vi "DO Close.vi"(8 "error in (no error)":errorcluster, 11 "Binary Valve in":refnum<class "Binary Valve.lvclass">) -> (0 "error out":errorcluster)   [LabVIEW 2021, in "Binary Valve.lvlib" / "Binary Valve.lvclass"]
uses:
  Binary Valve.lvclass
  Binary Valve.lvclass/Binary Valve.ctl
  <vilib>/NathanCo/Digital Tasks/Digital Output/Digital Output/Digital Output.lvclass
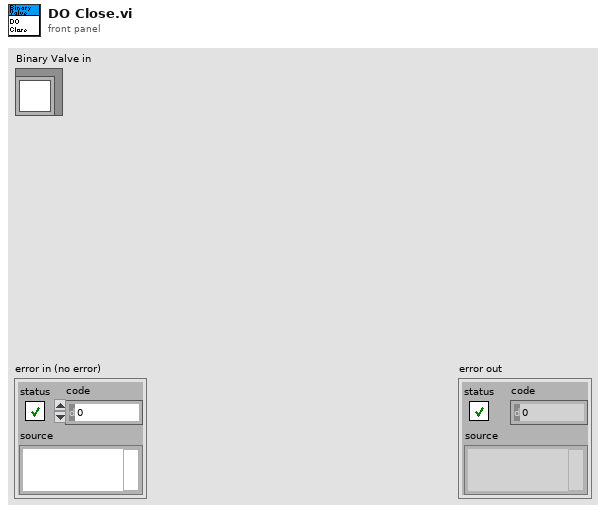
[diagram p1: front panel]
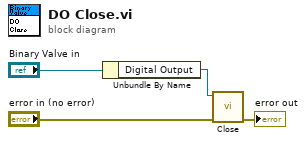
[diagram p0: block diagram]
diagram:
  n1 = Unbundle By Name("Binary Valve in") -> ("Digital Output"=w3:refnum<class "Digital Output.lvclass">)
  n2 = call <vilib>:"Close.vi"("error in (no error)"="error in (no error)", "Digital Output in"=w3) -> ("error out"=→"error out":errorcluster)  [unwired: 9 in]
